vi "Configure OVP.vi"(7 "Enable OVP (T: Enable)":bool=TRUE, 8 "error in (no error)":errorcluster, 9 "Voltage Limit (50.0 V)":dbl=50.0 format="%.2g", 11 "VISA resource name":refnum<visa-resource-name>) -> (0 "error out":errorcluster, 3 "VISA resource name out":refnum<visa-resource-name>)   [LabVIEW 2015, in "IT6700H.lvlib"]
doc: "Configures over voltage protection (OVP) of the power supply. Specify the voltage limit and whether to enable or disable OVP."
uses:
  <instrlib>/IT6700H/IT6700H.lvlib
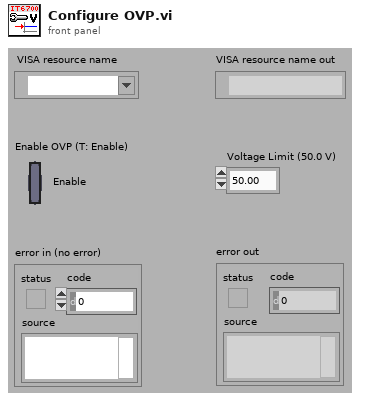
[diagram p1: front panel]
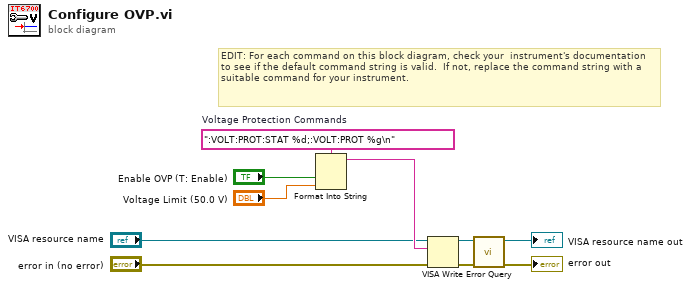
[diagram p0: block diagram]
diagram:
  w8 = ":VOLT:PROT:STAT %d;:VOLT:PROT %g\n"  # Voltage Protection Commands
  # "EDIT: For each command on this block diagram, check your  instrument's documentation to see if the default command string is valid.  If not, replace the command string with a suitable command for your instrument."
  n1 = Format Into String(format string=w8, "Enable OVP (T: Enable)", "Voltage Limit (50.0 V)") -> (resulting string=w5:string)  [unwired: 2 in, 1 out]
  n2 = VISA Write(VISA resource name="VISA resource name", write buffer=w5, error in (no error)="error in (no error)") -> (VISA resource name out=w6:refnum<visa-resource-name>, error out=w7:errorcluster)  [unwired: 1 out]
  n3 = call <instrlib>:"Error Query.vi"("error in (no error)"=w7, "VISA resource name"=w6) -> ("error out"=→"error out":errorcluster, "VISA resource name out"=→"VISA resource name out":refnum<visa-resource-name>)  [unwired: 6 in, 2 out]
